vi "tearDown.vi"(8 "error in (no error)":errorcluster, 11 "reference in":refnum<class "Engine Simulation IO System Tests.lvclass">) -> (0 "error out":errorcluster, 3 "reference out":refnum<class "Engine Simulation IO System Tests.lvclass">)   [LabVIEW 2015, in "Engine Simulation IO System Tests.lvclass"]
doc: "tearDown runs after the test method has completed. Use this method to clean up any operations or references that were opened by setUp or the test method. Unit tests should be independent of other unit tests so this VI should ensure that the next test can run in a 'clean' test environment."
uses:
  Engine Simulation IO System Tests.lvclass
  Engine Simulation IO System Tests.lvclass/Engine Simulation IO System Tests.ctl
  <vilib>/FPGAPlugInAG/Dynamic/niLvFpga_Close_Dynamic.vi
  <vilib>/rvi/interface/nirviCloseFPGA/nirviCloseFPGA.xnode
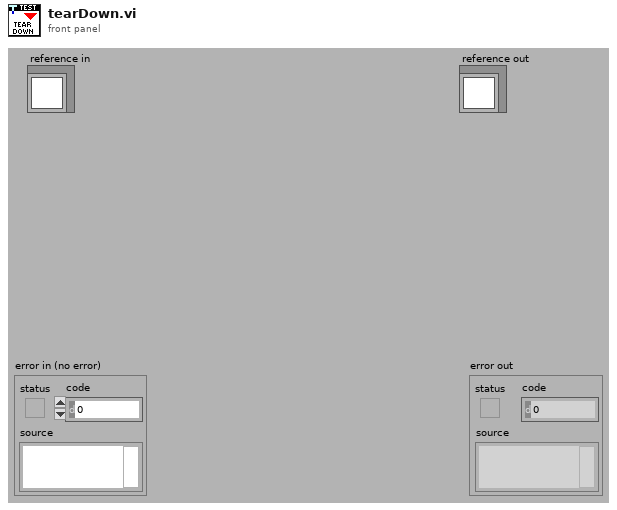
[diagram p1: front panel]
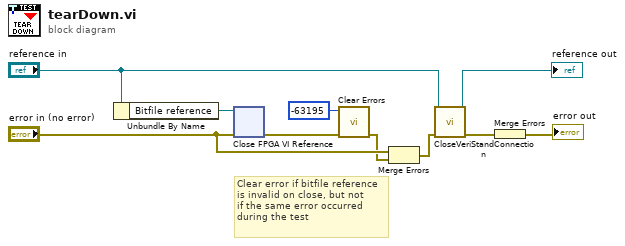
[diagram p0: block diagram]
diagram:
  # "Clear error if bitfile reference\nis invalid on close, but not\nif the same error occurred\nduring the test"
  n1 = Unbundle By Name("reference in") -> ("Bitfile reference"=w9:refnum<k20>)
  n2 = xnode "Close FPGA VI Reference"("FPGA VI Reference In"=w9, "error in"="error in (no error)") -> ("error out"=w8:errorcluster)
  n3 = call <vilib>:"Clear Errors.vi"("error in (no error)"=w8, "specific error code to clear (0: all)"=-63195) -> ("error out"=w2:errorcluster)  [unwired: 4 in, 1 out]
  n4 = Merge Errors("error in (no error)", w2) -> (w1:errorcluster)
  n5 = call-dynamic "CloseVeriStandConnection.vi"("error in (no error)"=w1, "VeriStand Test Case in"="reference in") -> ("error out"=w7:errorcluster, "VeriStand Test Case out"=→"reference out":refnum<class "Engine Simulation IO System Tests.lvclass">)  [unwired: 8 in]
  n6 = Merge Errors(w7) -> (→"error out":errorcluster)
